vi "Serialize Core.vi"(8 "error in":errorcluster, 10 "StrIn":string="{", 11 "variant":variant) -> (0 "error out":errorcluster, 1 "values":string[](array[string]), 2 "StrOut":string, 3 "Variant":variant)   [LabVIEW 2015, in "CVT.lvclass"]
uses:
  CVT.lvclass
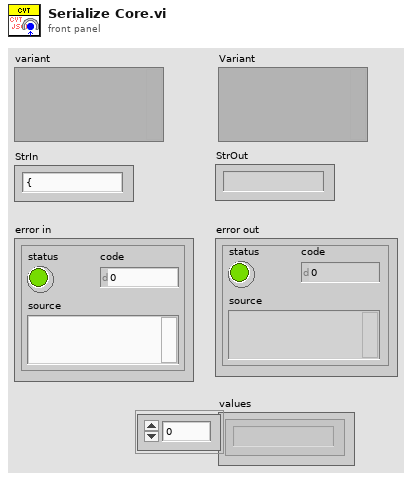
[diagram p1: front panel]
types:
  T1 = typedef "Type Descriptor Enumeration__ogtk.ctl" = enum8{"<Null>", "I8", "I16", "I32", "I64", "U8", "U16", "U32", "U64", "SGL", "DBL", "EXT", "CSG", "CDB", "CXT", "0x0F", "0x10", "0x11", "0x12", "0x13", "0x14", "Enum U8", "Enum U16", "Enum U32", "Enum U64", "SGL PQ", "DBL PQ", "EXT PQ", "CSG PQ", "CDB PQ", "CXT PQ", "0x1F", "0x20", "Boolean", "0x22", "0x23", "0x24", "0x25", "0x26", "0x27", "0x28", "0x29", "0x2A", "0x2B", "0x2C", "0x2D", "0x2E", "0x2F", "String", "0x31", "Path", "Pict", "0x34", "0x35", "0x36", "DAQ", "0x38", "0x39", "0x3A", "0x3B", "0x3C", "0x3D", "0x3E", "0x3F", "Array", "0x41", "0x42", "0x43", "0x44", "0x45", "0x46", "0x47", "0x48", "0x49", "0x4A", "0x4B", "0x4C", "0x4D", "0x4E", "0x4F", "Cluster", "0x51", "0x52", "Variant", "Waveform", "0x55", "0x56", "0x57", "0x58", "0x59", "0x5A", "0x5B", "0x5C", "0x5D", "0x5E", "0x5F", "0x60", "0x61", "0x62", "0x63", "0x64", "0x65", "0x66", "0x67", "0x68", "0x69", "0x6A", "0x6B", "0x6C", "0x6D", "0x6E", "0x6F", "Refnum"}
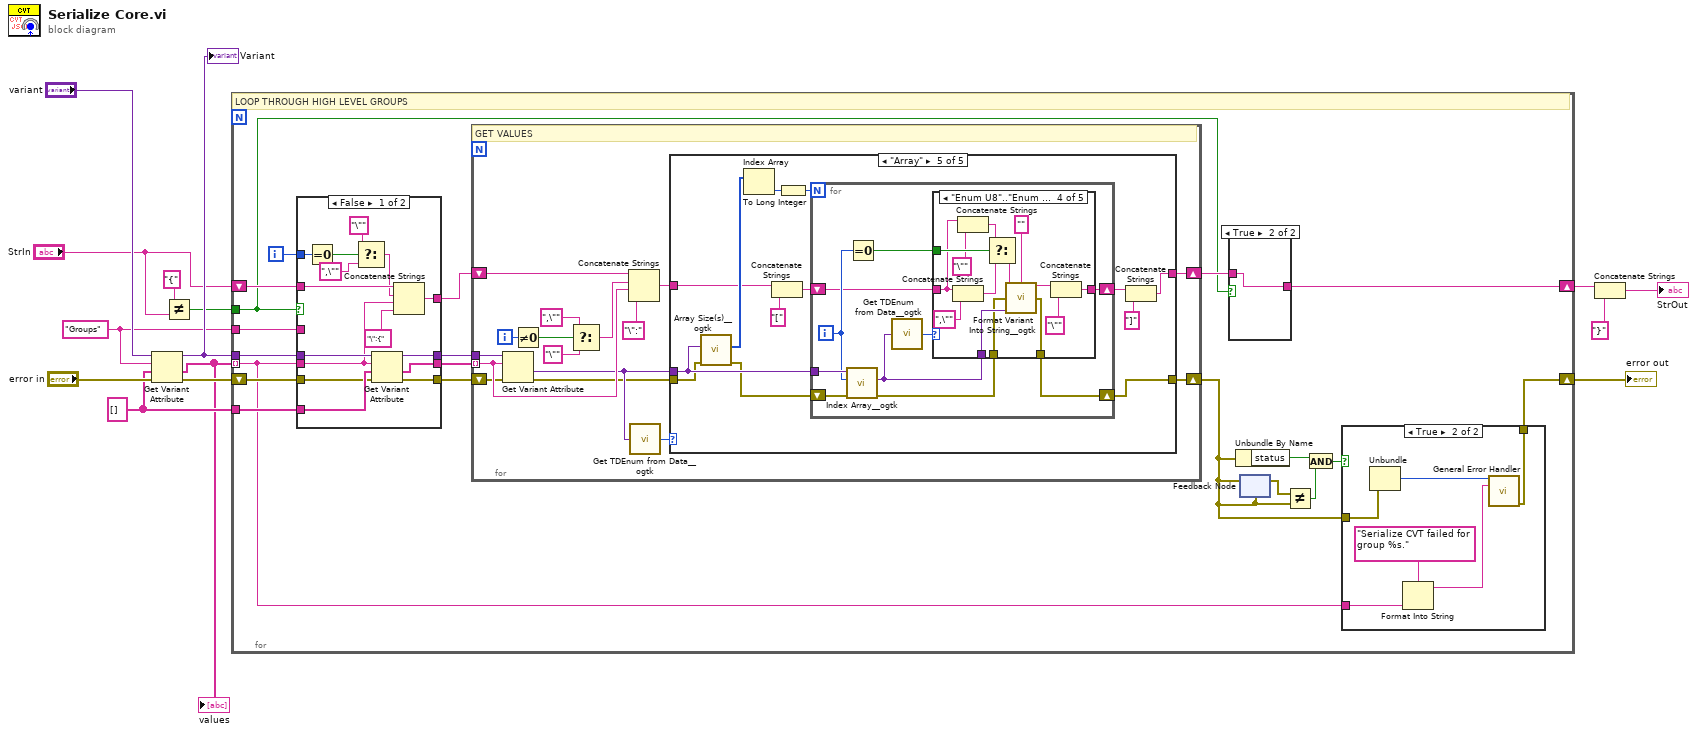
[diagram p0: block diagram]
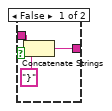
[diagram p3: hidden frame]
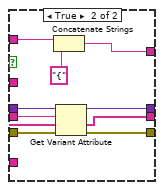
[diagram p4: hidden frame]
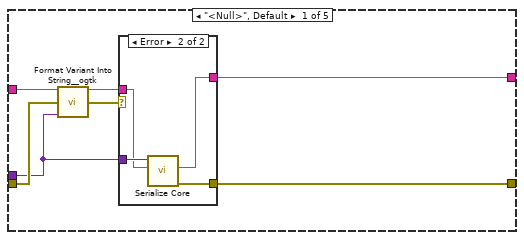
[diagram p5: hidden frame]
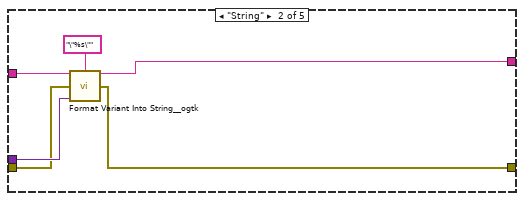
[diagram p7: hidden frame]
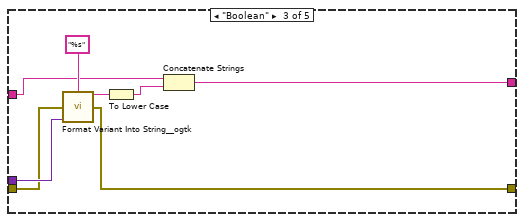
[diagram p8: hidden frame]
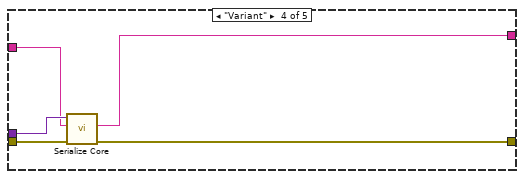
[diagram p9: hidden frame]
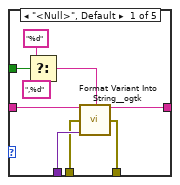
[diagram p10: hidden frame]
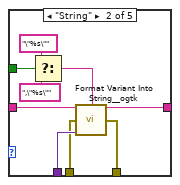
[diagram p11: hidden frame]
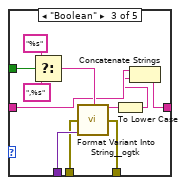
[diagram p12: hidden frame]
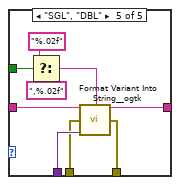
[diagram p13: hidden frame]
diagram:
  w7 = string[] []
  w2 = "Groups" ("name")
  n1 = Get Variant Attribute(Variant="variant", name=w2, default value (empty Variant)=w7, error in="error in") -> (duplicate Variant=w10:variant, value=w6:string[], error out=w13:errorcluster)  [unwired: 1 out]
  "Variant" <- w10
  "values" <- w6
  n2 = Not Equal?(x="{", y="StrIn") -> (x != y?=w1:bool)
  n3 = for {
    tunnel: w10 -> [w34]
    tunnel: w6 -> [w17] mode=indexing
    tunnel: w7 -> [w33]
    shift-right: [w26] -> w8
    shift-left: "StrIn" -> [w30]
    shift-right: [w15] -> w14
    shift-left: w13 -> [w25]
    tunnel: w1 -> [w22]
    tunnel: w2 -> [w23]
    i -> [w28]
    # "LOOP THROUGH HIGH LEVEL GROUPS"
    n4 = case shown="False" w22 {
      tunnel: w34 -> [w60 w70]
      tunnel: w33 -> [w59 w68]
      tunnel: [w58 w65] -> w32
      tunnel: [w57 w69] -> w31
      tunnel: w30 -> [w56 w63]
      tunnel: w17 -> [w55 w64]
      tunnel: [w53 w61] -> w29
      tunnel: w28 -> [w52 _]
      tunnel: w25 -> [w47 w67]
      tunnel: [w46 w66] -> w24
      tunnel: w23 -> [_ _]
      frame False {
        n5 = Equal To 0?(x=w52) -> (x = 0?=w51:bool)
        n6 = Select(t="\"" ("string"), s=w51, f=",\"" ("string")) -> (s? t:f=w48:string)
        n7 = Get Variant Attribute(Variant=w60, name=w55, default value (empty Variant)=w59, error in=w47) -> (duplicate Variant=w57:variant, value=w58:string[], error out=w46:errorcluster)  [unwired: 1 out]
        n8 = Concatenate Strings(w56, w48, w55, "\":{" ("string")) -> (w53:string)
      }
      frame True {
        n9 = Concatenate Strings(w63, "{" ("x")) -> (w61:string)
        n10 = Get Variant Attribute(Variant=w70, name=w64, default value (empty Variant)=w68, error in=w67) -> (duplicate Variant=w69:variant, value=w65:string[], error out=w66:errorcluster)  [unwired: 1 out]
      }
    }
    n11 = for {
      tunnel: w32 -> [w85] mode=indexing
      tunnel: w31 -> [w86]
      shift-right: [w75] -> w27
      shift-left: w29 -> [w83]
      shift-right: [w71] -> w16
      shift-left: w24 -> [w73]
      i -> [w82]
      # "GET VALUES"
      n12 = Get Variant Attribute(Variant=w86, name=w85, error in=w73) -> (value=w76:variant, error out=w72:errorcluster)  [unwired: 1 in, 2 out]
      n13 = Not Equal To 0?(x=w82) -> (x != 0?=w81:bool)
      n14 = Select(t=",\"" ("string"), s=w81, f="\"" ("string")) -> (s? t:f=w78:string)
      n15 = Concatenate Strings(w83, w78, w85, "\":" ("string")) -> (w74:string)
      n16 = call <userlib>:"Get TDEnum from Data__ogtk.vi"("Data"=w76) -> ("Type Descriptor Enumeration"=w77:T1)  [unwired: 4 in]
      n17 = case shown="\"Array\"" w77 {
        tunnel: w76 -> [w89 w105 w113 w118 w124]
        tunnel: [w90 w102 w106 w116 w126] -> w75
        tunnel: w74 -> [w93 w103 w107 w114 w130]
        tunnel: w72 -> [w92 w100 w110 w117 w123]
        tunnel: [w87 w101 w111 w115 w121] -> w71
        frame "<Null>", Default {
          n18 = call <userlib>:"Format Variant Into String__ogtk.vi"("Input String"=w93, "error in (no error)"=w92, "Variant"=w89) -> ("Output String"=w91:string, "error out"=w88:errorcluster)  [unwired: 11 in]
          n19 = case shown="Error" w88 {
            selector: w88 -> [w94 _]
            tunnel: w91 -> [w95 w97]
            tunnel: [w95 w96] -> w90
            tunnel: w89 -> [_ w99]
            tunnel: [w94 w98] -> w87
            frame No Error {
            }
            frame Error {
              n20 = call "Serialize Core.vi"("StrIn"=w97, "variant"=w99) -> ("error out"=w98:errorcluster, "StrOut"=w96:string)  [unwired: 6 in, 2 out]
            }
          }
        }
        frame "String" {
          n21 = call <userlib>:"Format Variant Into String__ogtk.vi"("Input String"=w103, "Format String"="\"%s\"", "error in (no error)"=w100, "Variant"=w105) -> ("Output String"=w102:string, "error out"=w101:errorcluster)  [unwired: 10 in]
        }
        frame "Boolean" {
          n22 = call <userlib>:"Format Variant Into String__ogtk.vi"("Format String"="%s", "error in (no error)"=w110, "Variant"=w113) -> ("Output String"=w109:string, "error out"=w111:errorcluster)  [unwired: 11 in]
          n23 = To Lower Case(string=w109) -> (all lower case string=w108:string)
          n24 = Concatenate Strings(w107, w108) -> (w106:string)
        }
        frame "Variant" {
          n25 = call "Serialize Core.vi"("error in"=w117, "StrIn"=w114, "variant"=w118) -> ("error out"=w115:errorcluster, "StrOut"=w116:string)  [unwired: 5 in, 2 out]
        }
        frame "Array" {
          n26 = call <userlib>:"Array Size(s)__ogtk.vi"("error in (no error)"=w123, "Array"=w124) -> ("error out"=w122:errorcluster, "Size(s)"=w131:u32[])  [unwired: 7 in, 1 out]
          n27 = Index Array(array=w131) -> (element=w120:u32)  [unwired: 1 in]
          n28 = Concatenate Strings(w130, "[" ("string")) -> (w128:string)
          n29 = To Long Integer(number=w120) -> (32bit integer=w119:i32)
          n30 = for {
            N: w119 -> [_]
            tunnel: w124 -> [w141]
            shift-right: [w135] -> w127
            shift-left: w128 -> [w136]
            shift-right: [w132] -> w121
            shift-left: w122 -> [w137]
            i -> [w140]
            n31 = call <userlib>:"Index Array__ogtk.vi"("error in (no error)"=w137, "Index (1D)"=w140, "MultiD Array"=w141) -> ("error out"=w133:errorcluster, "Array Element"=w134:variant)  [unwired: 7 in]
            n32 = Equal To 0?(x=w140) -> (x = 0?=w139:bool)
            n33 = call <userlib>:"Get TDEnum from Data__ogtk.vi"("Data"=w134) -> ("Type Descriptor Enumeration"=w138:T1)  [unwired: 4 in]
            n34 = case shown="\"Enum U8\"..\"Enum U32\"" w138 {
              tunnel: w139 -> [w148 w157 w168 w184 w193]
              tunnel: w136 -> [w146 w155 w162 w180 w189]
              tunnel: [w144 w153 w160 w174 w187] -> w135
              tunnel: w134 -> [w145 w154 w165 w173 w188]
              tunnel: w133 -> [w143 w152 w164 w172 w186]
              tunnel: [w142 w151 w163 w171 w185] -> w132
              frame "<Null>", Default {
                n35 = Select(t="%d", s=w148, f=",%d") -> (s? t:f=w147:string)
                n36 = call <userlib>:"Format Variant Into String__ogtk.vi"("Input String"=w146, "Format String"=w147, "error in (no error)"=w143, "Variant"=w145) -> ("Output String"=w144:string, "error out"=w142:errorcluster)  [unwired: 10 in]
              }
              frame "String" {
                n37 = Select(t="\"%s\"", s=w157, f=",\"%s\"") -> (s? t:f=w156:string)
                n38 = call <userlib>:"Format Variant Into String__ogtk.vi"("Input String"=w155, "Format String"=w156, "error in (no error)"=w152, "Variant"=w154) -> ("Output String"=w153:string, "error out"=w151:errorcluster)  [unwired: 10 in]
              }
              frame "Boolean" {
                n39 = Select(t="%s", s=w168, f=",%s") -> (s? t:f=w167:string)
                n40 = call <userlib>:"Format Variant Into String__ogtk.vi"("Format String"=w167, "error in (no error)"=w164, "Variant"=w165) -> ("Output String"=w166:string, "error out"=w163:errorcluster)  [unwired: 11 in]
                n41 = To Lower Case(string=w166) -> (all lower case string=w161:string)
                n42 = Concatenate Strings(w162, w161) -> (w160:string)
              }
              frame "Enum U8".."Enum U32" {
                n43 = Concatenate Strings(w180, ",\"" ("string")) -> (w182:string)
                n44 = Concatenate Strings(w180, "\"" ("string")) -> (w181:string)
                n45 = Select(t=w181, s=w184, f=w182) -> (s? t:f=w177:string)
                n46 = call <userlib>:"Format Variant Into String__ogtk.vi"("Input String"=w177, "Format String"="", "error in (no error)"=w172, "Variant"=w173) -> ("Output String"=w175:string, "error out"=w171:errorcluster)  [unwired: 10 in]
                n47 = Concatenate Strings(w175, "\"" ("string")) -> (w174:string)
              }
              frame "SGL", "DBL" {
                n48 = Select(t="%.02f", s=w193, f=",%.02f") -> (s? t:f=w190:string)
                n49 = call <userlib>:"Format Variant Into String__ogtk.vi"("Input String"=w189, "Format String"=w190, "error in (no error)"=w186, "Variant"=w188) -> ("Output String"=w187:string, "error out"=w185:errorcluster)  [unwired: 10 in]
              }
            }
          }
          n50 = Concatenate Strings(w127, "]" ("string")) -> (w126:string)
        }
      }
    }
    n51 = case shown="True" w22 {
      tunnel: w27 -> [w44 w45]
      tunnel: [w42 w45] -> w26
      frame False {
        n52 = Concatenate Strings(w44, "}" ("string")) -> (w42:string)
      }
      frame True {
      }
    }
    n53 = Unbundle By Name(w16) -> ("status"=w19:bool)
    n54 = feedback-in #1(w16) -> ()
    n55 = feedback #1(w16) -> (w21:errorcluster)
    n56 = Not Equal?(x=w21, y=w16) -> (x != y?=w20:bool)
    n57 = And(x=w19, y=w20) -> (x .and. y?=w18:bool)
    n58 = case shown="True" w18 {
      tunnel: w16 -> [w35 w41]
      tunnel: w17 -> [_ w39]
      tunnel: [w35 w36] -> w15
      frame False {
      }
      frame True {
        n59 = Unbundle(w41) -> ("code"=w40:i32)  [unwired: 2 out]
        n60 = Format Into String(format string="Serialize CVT failed for group %s.", w39) -> (resulting string=w37:string)  [unwired: 2 in, 1 out]
        n61 = call <vilib>:"General Error Handler.vi"("[error code] (0)"=w40, "[error source] (\" \")"=w37) -> ("error out"=w36:errorcluster)  [unwired: 9 in, 4 out]
      }
    }
  }
  "error out" <- w14
  n62 = Concatenate Strings(w8, "}" ("string")) -> (→"StrOut":string)
